vi "ArrayFunctions_CheckForDups(String).vi"(1 "Array":string[](array[string])) -> (15 "DupElements":string[](array[string]), 16 "DupElements(String)":string, 17 "FoundDups":bool)   [LabVIEW 2016]
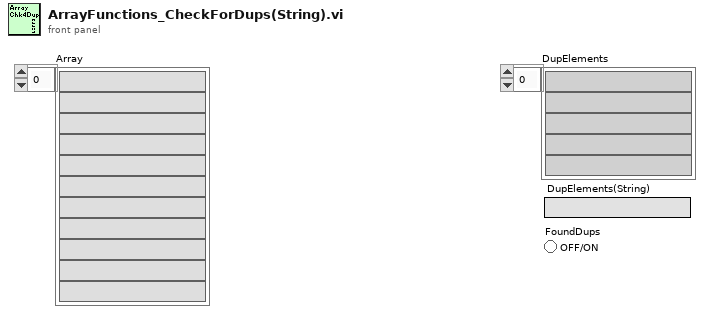
[diagram p1: front panel]
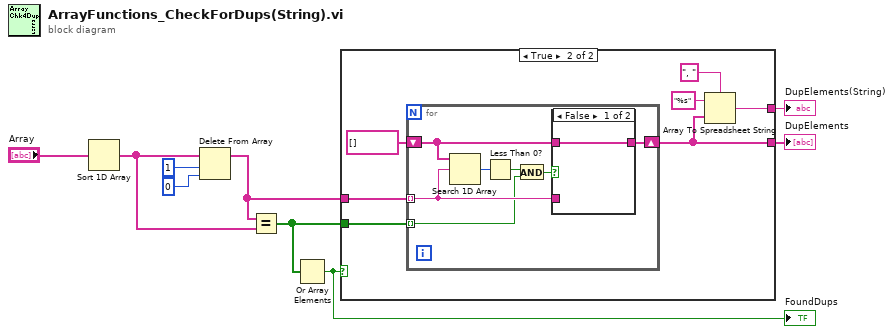
[diagram p0: block diagram]
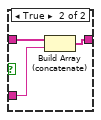
[diagram p3: hidden frame]
diagram:
  n1 = Sort 1D Array(array="Array") -> (sorted array=w2:string[])
  n2 = Delete From Array(array=w2, length=1, index=0) -> (array with subset deleted=w7:string[])  [unwired: 1 out]
  n3 = Equal?(x=w7, y=w2) -> (x = y?=w6:bool[])
  n4 = Or Array Elements(Boolean array=w6) -> (logical OR=w4:bool)
  "FoundDups" <- w4
  n5 = case shown="True" w4 {
    tunnel: w7 -> [_ w16]
    tunnel: w6 -> [_ w15]
    tunnel: [_ w13] -> w5
    tunnel: [_ w10] -> w1
    frame False {
    }
    frame True {
      n6 = for {
        tunnel: w16 -> [w21] mode=indexing
        tunnel: w15 -> [w17] mode=indexing
        shift-right: [w23] -> w13
        shift-left: string[] [] ("array w/ subset deleted") -> [w22]
        n7 = Search 1D Array(1D array=w22, element=w21) -> (index of element=w20:i32)  [unwired: 1 in]
        n8 = Less Than 0?(x=w20) -> (x < 0?=w19:bool)
        n9 = And(x=w19, y=w17) -> (x .and. y?=w18:bool)
        n10 = case shown="False" w18 {
          tunnel: [w24 w27] -> w23
          tunnel: w22 -> [w24 w26]
          tunnel: w21 -> [_ w25]
          frame False {
          }
          frame True {
            n11 = Build Array (concatenate)(w26, w25) -> (w27:string[])
          }
        }
      }
      n12 = Array To Spreadsheet String(delimiter (Tab)=", ", array=w13, 3:"%s" ("format string")) -> (spreadsheet string=w10:string)
    }
  }
  "DupElements" <- w5
  "DupElements(String)" <- w1
